vi "GetSet_TS_Step_Param_LV2015.vi"(7 "Sequence Context In":refnum<k7>, 8 "error in":errorcluster, 10 "GET?":bool, 11 "Parameters In":cluster{"Numeric":dbl, "String":string}) -> (0 "error out":errorcluster, 3 "Parameters Out":cluster{"Numeric":dbl, "String":string})   [LabVIEW 2015]
doc: "This VI sets or gets the TTI_CPX400DP PSU settings.\nCreated By Shane Donnellan\n\n<b> Get </B> Allows the system to set or set the TS variables.\n\n\n<b>Visa resourses</B> The resourse i.e. the GPIB port use the device manager to locate the PSU.\n\n<b>Channel</B> The Channel to use on the PSU.\n\n<B>Actions</B> The Actions the PSU will under take.\n<B>Reset</B> Reset the PSU \n<b>Set Channel</B> Set the Channel Active.\n<B>Measure</B> Measure the Current and Voltage.\n\n<b>Volage (V)</B> The Volage to set the PSU to.\n<b>Current Limit (A)</b> The PSU Current Limit.\n<B>OVP Limit (V)</b> The Over Voltage Protection Limit in volts.\n<B>Output</B> The Output of the system to On Off\n\n\n<B>Act Voltage</B> The Actual Voltage of the PSU the Value recorded by the PSU.\n<B>Act Current (A)</B> The Actual Current of the PSU the Value recorded by the PSU.\n<B>Act Power</B> The Act Power of the PSU the Value recorded by the PSU."
panel:
  # "Connector Pane"
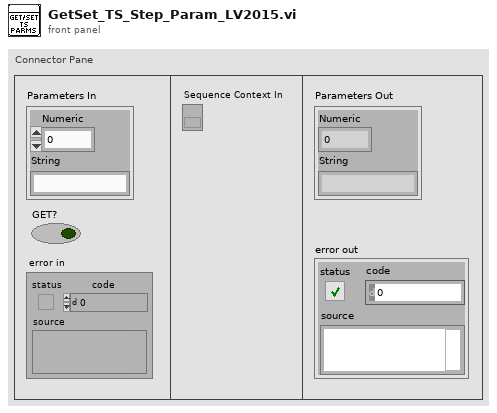
[diagram p1: front panel]
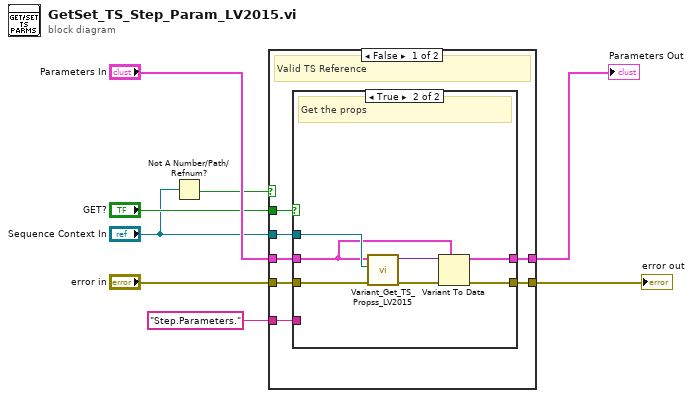
[diagram p0: block diagram]
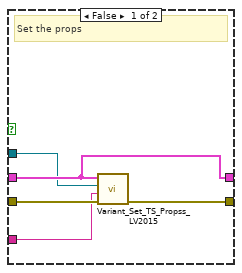
[diagram p2: hidden frame]
diagram:
  n1 = Not A Number/Path/Refnum?(number/path/refnum="Sequence Context In") -> (NaN/Path/Refnum?=w3:bool)
  n2 = case shown="False" w3 {
    tunnel: "GET?" -> [w15 _]
    tunnel: "Parameters In" -> [w14 w29]
    tunnel: [w13 w29] -> w4
    tunnel: "error in" -> [w12 w28]
    tunnel: [w11 w28] -> w2
    tunnel: "Sequence Context In" -> [w10 _]
    tunnel: "Step.Parameters." -> [w9 _]
    frame False {
      # "Valid TS Reference"
      n3 = case shown="True" w15 {
        tunnel: w14 -> [w18 w21]
        tunnel: [w18 w22] -> w13
        tunnel: w12 -> [w20 w27]
        tunnel: [w19 w24] -> w11
        tunnel: w10 -> [w17 w25]
        tunnel: w9 -> [w16 _]
        frame False {
          # "Set the props"
          n4 = call "Variant_Set_TS_Propss_LV2015.vi"("error in (no error)"=w20, "TS Paramter Ref Str"=w16, "Sequence Context In"=w17, "Parameters In"=w18) -> ("error out"=w19:errorcluster)  [unwired: 6 in, 1 out]
        }
        frame True {
          # "Get the props"
          n5 = call "Variant_Get_TS_Propss_LV2015.vi"("error in (no error)"=w27, "Sequence Context In"=w25, "Variant (Type) In"=w21) -> ("error out"=w26:errorcluster, "Variant of Input Type"=w23:variant)  [unwired: 7 in]
          n6 = Variant To Data(error in=w26, type=w21, Variant=w23) -> (data=w22:cluster{"Numeric":dbl, "String":string}, error out=w24:errorcluster)
        }
      }
    }
    frame True {
    }
  }
  "Parameters Out" <- w4
  "error out" <- w2
